vi "Windows_Get Font Name Array.vi"(8 "Error":errorcluster) -> (0 "Error Out":errorcluster, 3 "Windows Font Array Out":string[](array[string]))   [LabVIEW 2021]
uses:
  <vilib>/registry/registry.llb/Registry SAM.ctl
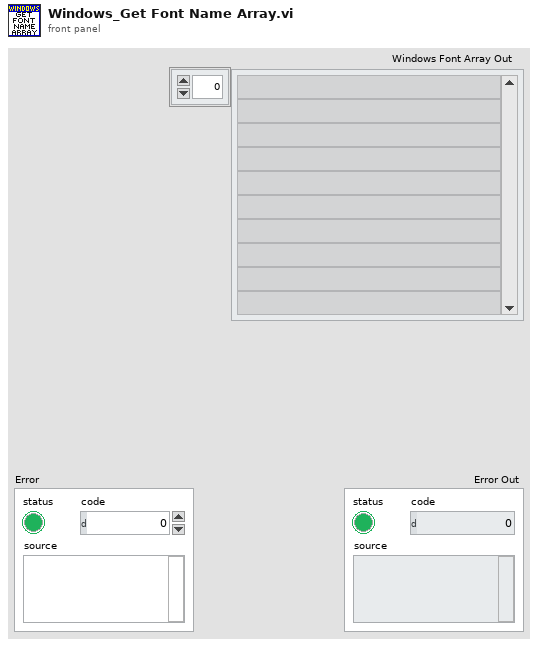
[diagram p1: front panel]
types:
  T1 = typedef "Registry SAM.ctl" = enum32{"KEY_QUERY_VALUE", "KEY_SET_VALUE", "KEY_CREATE_SUB_KEY", "KEY_ENUMERATE_SUB_KEYS", "KEY_NOTIFY", "KEY_CREATE_LINK", "KEY_READ", "KEY_WRITE", "KEY_ALL_ACCESS", "KEY_READ | KEY_WRITE"}
  T2 = typedef "Registry refnum.ctl" = refnum<k1>
  T3 = cluster{"numValues":i32, "maxValueNameLen":i32, "maxValueDataLen":i32}
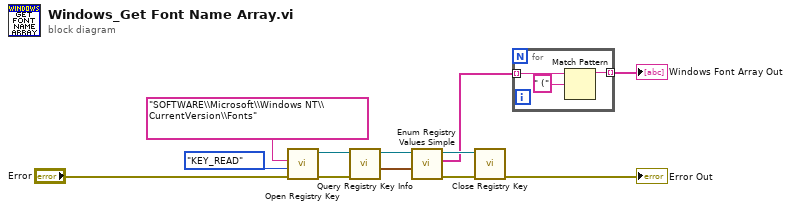
[diagram p0: block diagram]
diagram:
  n1 = call <vilib>:"Open Registry Key.vi"("error in (no error)"="Error", "security access mask (KEY_READ | KEY_WRITE)"=Registry_SAM."KEY_READ", "subkey"="SOFTWARE\\Microsoft\\Windows NT\\CurrentVersion\\Fonts") -> ("error out"=w9:errorcluster, "refnum out"=w10:T2)  [unwired: 1 in, 6 out]
  n2 = call <vilib>:"Query Registry Key Info.vi"("error in (no error)"=w9, "refnum"=w10) -> ("value info"=w8:T3, "refnum out"=w7:T2)  [unwired: 8 out]
  n3 = call <vilib>:"Enum Registry Values Simple.vi"("value info"=w8, "refnum"=w7) -> ("error out"=w6:errorcluster, "values"=w4:string[], "refnum out"=w5:T2)  [unwired: 2 in, 5 out]
  n4 = call <vilib>:"Close Registry Key.vi"("error in (no error)"=w6, "refnum"=w5) -> ("error out"=→"Error Out":errorcluster)  [unwired: 5 out]
  n5 = for {
    tunnel: w4 -> [w15] mode=indexing
    tunnel: [w13] -> w2 mode=indexing
    n6 = Match Pattern(string=w15, regular expression=" (") -> (before substring=w13:string)  [unwired: 4 out]
  }
  "Windows Font Array Out" <- w2
